vi "Save Config.vi"(8 "error in (no error)":errorcluster, 9 "Value in":variant, 10 "Section":string, 11 "Project in":refnum<class "Project.lvclass">) -> (0 "error out":errorcluster, 3 "Project out":refnum<class "Project.lvclass">)   [LabVIEW 2015, in "Project.lvclass"]
uses:
  Project.lvclass
  <vilib>/Utility/config.llb/NI_LVConfig.lvlib
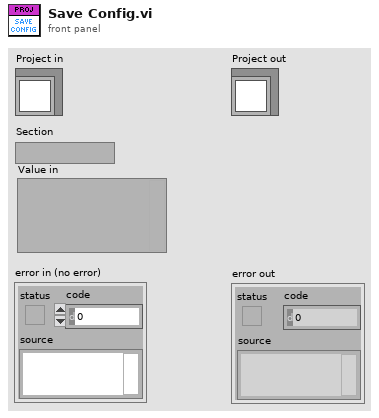
[diagram p1: front panel]
types:
  T1 = typedef "NI_LVConfig.lvlib/Config Data RefNum.ctl" = refnum<k1>
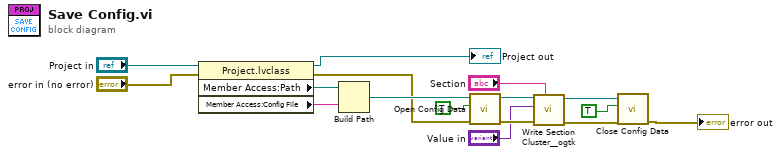
[diagram p0: block diagram]
diagram:
  n1 = property class="Project.lvclass"(reference="Project in", error in="error in (no error)") -> (reference out=→"Project out":refnum<class "Project.lvclass">, error out=w6:errorcluster, "Member Access:Path"=w9:path, "Member Access:Config File"=w8:string)
  n2 = Build Path(base path=w9, name or relative path=w8) -> (appended path=w7:path)
  n3 = call <vilib>:"Open Config Data.vi"("error in (no error)"=w6, "create file if necessary (T)"=TRUE, "configuration file path"=w7) -> ("error out"=w11:errorcluster, "refnum"=w12:T1)  [unwired: 6 in, 1 out]
  n4 = call <userlib>:"Write Section Cluster__ogtk.vi"("section (optional)"="Section", "error in (no error)"=w11, "Section Formatted Cluster"="Value in", "refnum"=w12) -> ("error out"=w13:errorcluster, "dup refnum"=w14:T1)  [unwired: 6 in]
  n5 = call <vilib>:"Close Config Data.vi"("error in (no error)"=w13, "write file if changed (T)"=TRUE, "refnum"=w14) -> ("error out"=→"error out":errorcluster)  [unwired: 7 in, 1 out]
